vi "tokenize_to_array.vi"(1 "File Contents":string) -> (0 "Lines":string[](array[string]))   [LabVIEW 2015]
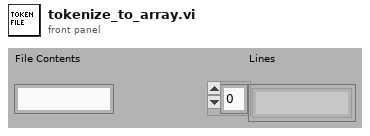
[diagram p1: front panel]
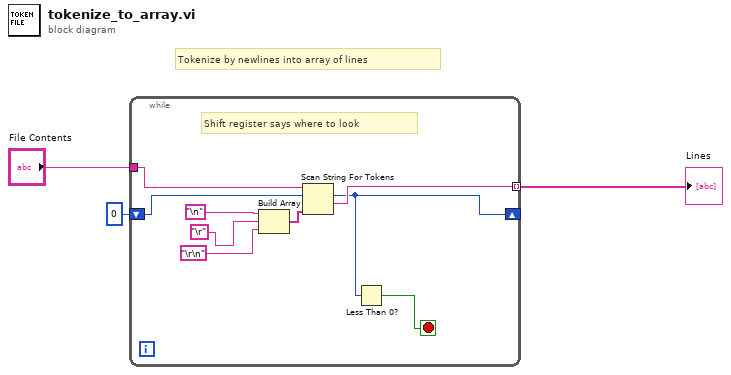
[diagram p0: block diagram]
diagram:
  # "Tokenize by newlines into array of lines"
  n1 = while {
    tunnel: "File Contents" -> [w12]
    shift-right: [w8] -> _
    shift-left: 0 ("offset past token") -> [w11]
    tunnel: [w9] -> w3 mode=indexing
    stop <- w10 stop-if-true
    # "Shift register says where to look"
    n2 = Build Array("\n", "\r", "\r\n") -> (w7:string[])
    n3 = Scan String For Tokens(6:w7, 8:w11, 9:w12) -> (1:w9:string, 2:w8:i32)  [unwired: 5 out]
    n4 = Less Than 0?(x=w8) -> (x < 0?=w10:bool)
  }
  "Lines" <- w3
